vi "Display Info.vi"(7 "Layout ref":refnum<vi>, 8 "error in (no error)":errorcluster, 9 "Modify (F) /Add [T]":bool, 10 "Names in use":string[](array[string]), 11 "Arduino DDS in":refnum<class "Arduino DDS.lvclass">) -> (0 "error out":errorcluster, 1 "Names in use out":string[](array[string]), 2 "Changes Made?":bool, 3 "Arduino DDS out":refnum<class "Arduino DDS.lvclass">)   [LabVIEW 2013, in "Arduino DDS.lvclass"]
uses:
  Arduino DDS.lvclass
  Device/Device.lvclass
panel:
  # "This VI just sets the wiring structure.\nOpen a child override version instead!"
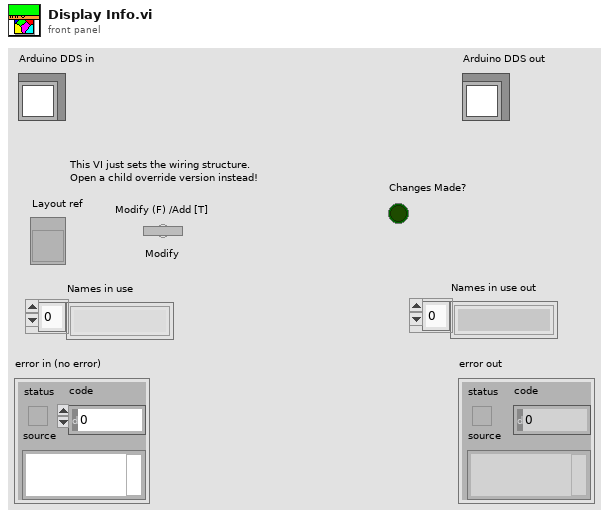
[diagram p1: front panel]
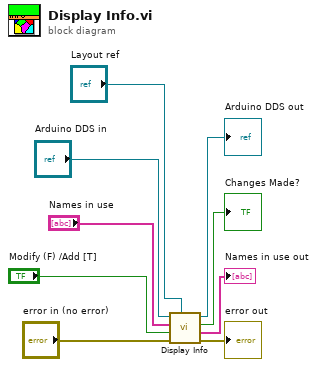
[diagram p0: block diagram]
diagram:
  n1 = call-parent "Display Info.vi"("Layout ref"="Layout ref", "error in (no error)"="error in (no error)", "Modify (F) /Add [T]"="Modify (F) /Add [T]", "Names in use"="Names in use", "Device in"="Arduino DDS in") -> ("error out"=→"error out":errorcluster, "Names in use out"=→"Names in use out":string[], "Changes Made?"=→"Changes Made?":bool, "Device out"=→"Arduino DDS out":refnum<class "Arduino DDS.lvclass">)  [unwired: 3 in]
